vi "Extract the Sine Wave - DFD.vi"() -> ()   [LabVIEW 2023]
doc: "Demonstrates how you can extract a signal from band-limited noise using VIs in the LabVIEW Digital Filter Design Toolkit."
uses:
  <vilib>/addons/Digital Filter Design/Process.llb/DFD Filtering (Array).vi
  <vilib>/Analysis/NI_AALBase.lvlib
  <vilib>/addons/Digital Filter Design/NI_DigFilterLicensed.lvlib
panel:
  in  "stop":bool
  in  "Filter Order":i32(slide)=5 scale=0.0..10.0
  in  "Cut-Off\nFrequency (Hz)":dbl(slide)=20.0 scale=0.0..50.0 scale format="%0.2f"
  in  "Sine Frequency (Hz)":dbl=10.0 format="%0.2f"
  out "?":cluster{dbl, dbl, dbl[]}(graph)={0.0, 0.001, []}
  out "?":cluster{dbl, dbl, dbl[]}(graph)={0.0, 0.001, []}
  # "Select Help»Show Context Help and move the cursor over the VI icon for more information."
  # "V"
  # "V"
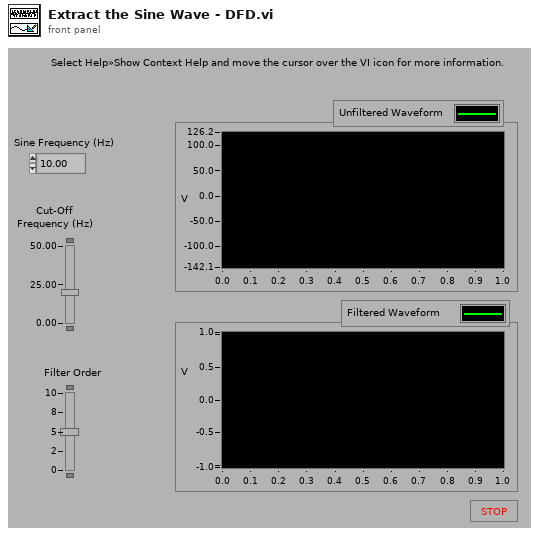
[diagram p1: front panel]
types:
  T1 = enum16{"Lowpass", "Highpass", "Bandpass", "Bandstop"}
  T2 = typedef "NI_DigFilterLicensed.lvlib/DFD Filter Obj.ctl" = cluster{"mSRate_Fs":dbl, "mSRate_Version":string, "mSRate_Comments":string, "mSRate_OrgCoef":T3, "mSRate_CurCoef":T3, "mSRate_Quantized?":bool, "mSRate_QCoef":T3, "mSRate_QSettings":T5[], "mSRate_Order":i32, "mSRate_Scaling":cluster{"mSRate_ScaleByPowerOf2?":bool, "mSRate_ScaleType":T7}}
  T3 = typedef "NI_DigFilterLicensed.lvlib/DFD Filter Coef.ctl" = cluster{"type":T4, "gain":dbl, "coef a (k)":dbl[], "coef b (v)":dbl[]}
  T4 = typedef "NI_DigFilterLicensed.lvlib/DFD Filter Structure Type Selector.ctl" = enum16{"Undefined", "FIR Direct Form", "FIR Direct Form Transposed", "FIR Symmetric", "FIR Antisymmetric", "IIR Direct Form I", "IIR Direct Form I Transposed", "IIR Direct Form II", "IIR Direct Form II Transposed", "IIR Cascaded Second Order Sections Form I", "IIR Cascaded Second Order Sections Form I Transposed", "IIR Cascaded Second Order Sections Form II", "IIR Cascaded Second Order Sections Form II Transposed", "Lattice Allpass (basic sections)", "Lattice Allpass (one multiplier sections)", "Lattice Allpass (normalized sections)", "Lattice AR (basic sections)", "Lattice AR (one multiplier sections)", "Lattice AR (normalized sections)", "Lattice MA (minimum phase)", "Lattice MA (maximum phase)", "Lattice ARMA (basic sections)", "Lattice ARMA (one multiplier sections)", "Lattice ARMA (normalized sections)"}
  T5 = typedef "NI_DigFilterLicensed.lvlib/dfd_Internal Quantization Settings.ctl" = cluster{"source":T6, "wl":i16, "iwl":i16, "overflow mode":enum16{"Saturation", "Wrap"}, "rounding mode":enum16{"Nearest", "Truncation"}, "signed?":bool}
  T6 = typedef "NI_DigFilterLicensed.lvlib/dfd_Internal Quantization Srcs.ctl" = u16
  T7 = typedef "NI_DigFilterLicensed.lvlib/DFD Coef Norm Type.ctl" = enum16{"No Norm", "Time Domain 1-Norm", "Time Domain 2-Norm", "Time Domain Inf-Norm"}
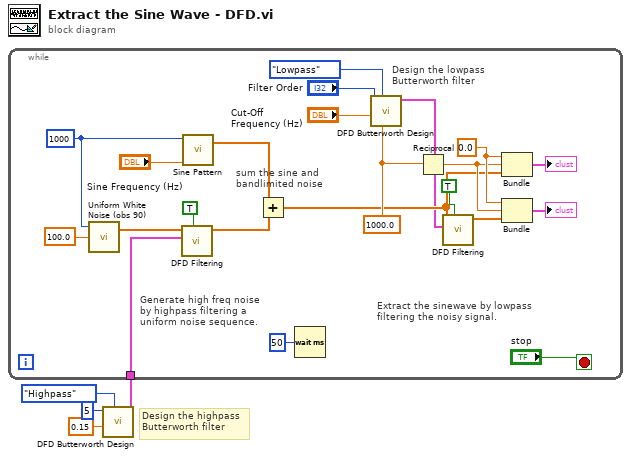
[diagram p0: block diagram]
diagram:
  # "Design the highpass\nButterworth filter"
  n1 = call <vilib>:"DFD Butterworth Design.vi"("filter type"=T1."Highpass", "low cutoff freq [Hz]"=0.15, "order"=5) -> ("filter out"=w1:T2)  [unwired: 3 in, 5 out]
  n2 = while {
    tunnel: w1 -> [w16]
    stop <- "stop" stop-if-true
    w23 = 0.0
    w9 = 1000.0
    w25 = 1000
    # "Design the lowpass\nButterworth filter"
    # "sum the sine and \nbandlimited noise"
    # "Extract the sinewave by lowpass\nfiltering the noisy signal."
    # "Generate high freq noise\nby highpass filtering a\nuniform noise sequence."
    n3 = call <vilib>:"Uniform White Noise (obs 90).vi"("amplitude"=100.0, "samples"=w25) -> ("uniform white noise"=w15:dbl[])  [unwired: 1 in, 1 out]
    n4 = call-poly <vilib>:"DFD Filtering.vi"("init? (F)"=TRUE, "filter"=w16, "signal in"=w15) -> ("signal out"=w14:dbl[])  [unwired: 1 in, 7 out]
    n5 = call <vilib>:"Sine Pattern.vi"("cycles"="Sine Frequency (Hz)", "samples"=w25) -> ("Sinusoidal Pattern"=w13:dbl[])  [unwired: 2 in, 1 out]
    n6 = Add(x=w13, y=w14) -> (x+y=w8:dbl[])
    n7 = Wait (ms)(milliseconds to wait=u32 50) -> ()  [unwired: 1 out]
    n8 = call <vilib>:"DFD Butterworth Design.vi"("fs [Hz]"=w9, "filter type"=T1."Lowpass", "low cutoff freq [Hz]"="Cut-Off\nFrequency (Hz)", "order"="Filter Order") -> ("filter out"=w7:T2)  [unwired: 2 in, 5 out]
    n9 = Reciprocal(x=w9) -> (1/x=w20:dbl)
    n10 = call-poly <vilib>:"DFD Filtering.vi"("init? (F)"=TRUE, "filter"=w7, "signal in"=w8) -> ("signal out"=w6:dbl[])  [unwired: 1 in, 7 out]
    n11 = Bundle(w23, w20, w8) -> (→"?":cluster{dbl, dbl, dbl[]})  [unwired: 1 out]
    n12 = Bundle(w23, w20, "signal out"=w6) -> (→"?":cluster{dbl, dbl, "signal out":dbl[]})  [unwired: 1 out]
  }
